vi "hbTest1.vi"() -> ()   [LabVIEW 2020]
uses:
  <vilib>/measure/mamon.llb/Waveform Peak Detection for N Chan.vi
  <vilib>/measure/NI_MAPro.lvlib
panel:
  out "Monitor Graph":dynamicdata(graph)
  in  "stop":bool
  out "BPM":dbl
  out "Frequency(Hz)":dbl
  out "Scalar":dbl
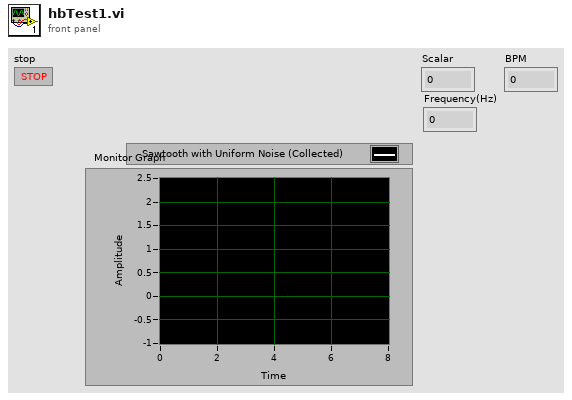
[diagram p1: front panel]
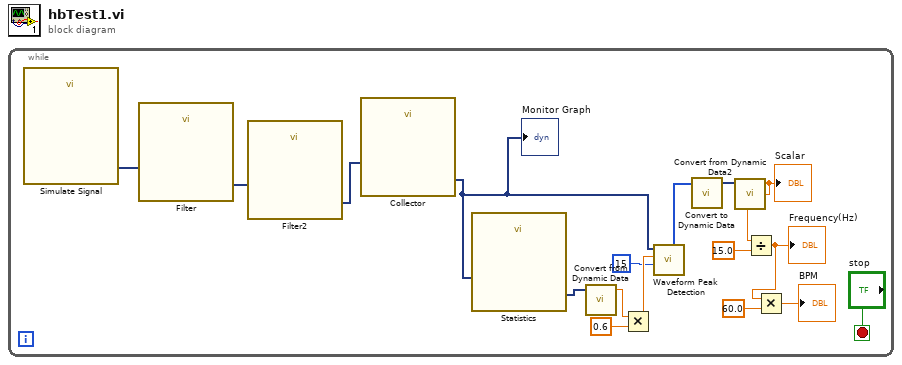
[diagram p0: block diagram]
diagram:
  n1 = while {
    stop <- "stop" stop-if-true
    n2 = call "Simulate Signal"() -> ("Sawtooth with Uniform Noise"=w17:dynamicdata)  [unwired: 14 in, 1 out]
    n3 = call "Filter"("Signal"=w17) -> ("Filtered Signal"=w16:dynamicdata)  [unwired: 9 in, 1 out]
    n4 = call "Filter2"("Signal"=w16) -> ("Filtered Signal"=w15:dynamicdata)  [unwired: 9 in, 1 out]
    n5 = call "Collector"("Signals"=w15) -> ("Collected Signals"=w1:dynamicdata)  [unwired: 9 in, 1 out]
    "Monitor Graph" <- w1
    n6 = call "Statistics"("Signals"=w1) -> ("Maximum"=w14:dynamicdata)  [unwired: 25 in, 1 out]
    n7 = call "Convert from Dynamic Data"("Dynamic Data Type"=w14) -> ("Scalar"=w12:dbl)  [unwired: 3 in]
    n8 = Multiply(x=w12, y=0.6) -> (x*y=w11:dbl)
    n9 = call-poly <vilib>:"Waveform Peak Detection.vi"("width"=15, "threshold"=w11, "Signals In"=w1) -> ("# found"=w9:i32[])  [unwired: 4 in, 4 out]
    n10 = call "Convert to Dynamic Data"("Array"=w9) -> ("Dynamic Data Type"=w8:dynamicdata)  [unwired: 3 in]
    n11 = call "Convert from Dynamic Data2"("Dynamic Data Type"=w8) -> ("Scalar"=w7:dbl)  [unwired: 3 in]
    "Scalar" <- w7
    n12 = Divide(x=w7, y=15.0) -> (x/y=w5:dbl)
    "Frequency(Hz)" <- w5
    n13 = Multiply(x=w5, y=60.0) -> (x*y=→"BPM":dbl)
  }
